vi "Fill Tree.vi"(8 "error in":errorcluster, 10 "Folder Path":path, 11 "TreeControl in":refnum<vi>) -> (0 "error out":errorcluster)   [LabVIEW 2019, in "SimpleDependencyInspector.lvlib" / "File Explorer.lvlib"]
uses:
  File Explorer.lvlib
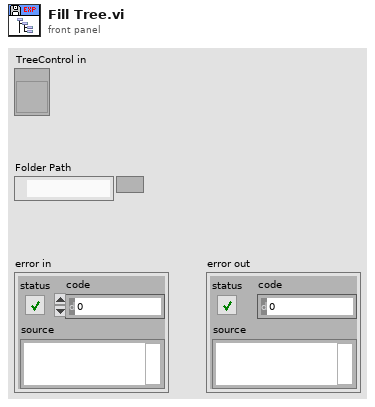
[diagram p1: front panel]
types:
  T1 = typedef "imagedata.ctl" = cluster{"image type":i32, "image depth":i32, "image":u8[], "mask":u8[], "colors":u32[], "Rectangle":cluster{"left":i16, "top":i16, "right":i16, "bottom":i16}}
  T2 = cluster{"Left Cell String":string, "Child Text":string[], "Child Tag":string, "Item Indent":i32, "Child Only?":bool, "Glyph Index":i32}[]
  T3 = cluster{"Left Cell String":string, "Child Text":string[], "Child Tag":string, "Item Indent":i32, "Child Only?":bool, "Glyph Index":i32}
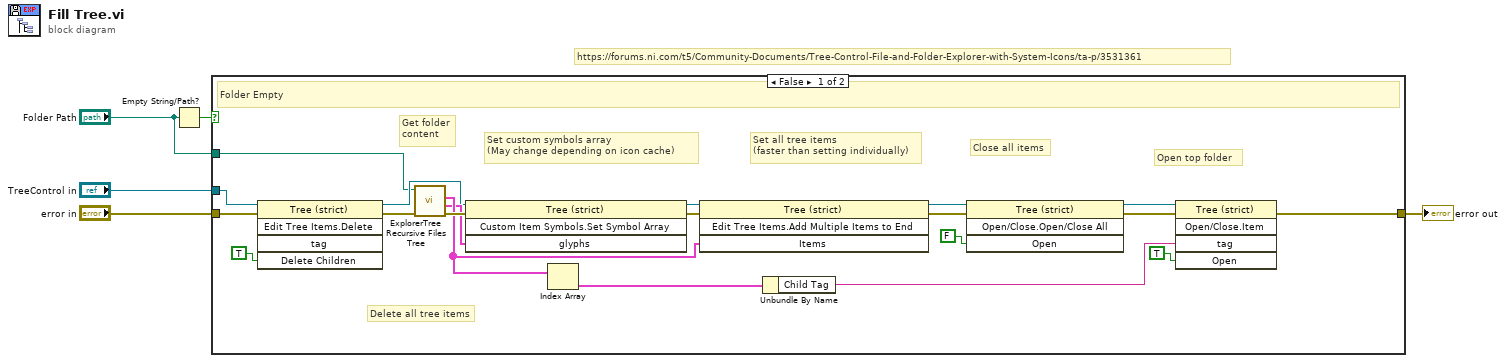
[diagram p0: block diagram]
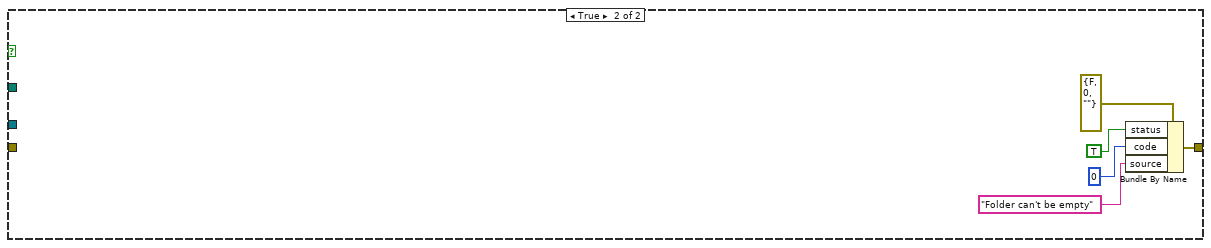
[diagram p2: hidden frame]
diagram:
  # "https://forums.ni.com/t5/Community-Documents/Tree-Control-File-and-Folder-Explorer-with-System-Icons/ta-p/3531361"
  n1 = Empty String/Path?(string/path="Folder Path") -> (empty?=w1:bool)
  n2 = case shown="False" w1 {
    tunnel: [w25 w29] -> w5
    tunnel: "error in" -> [w19 _]
    tunnel: "TreeControl in" -> [w7 _]
    tunnel: "Folder Path" -> [w6 _]
    frame False {
      # "Open top folder"
      # "Close all items"
      # "Set all tree items\n(faster than setting individually)"
      # "Set custom symbols array\n(May change depending on icon cache)"
      # "Get folder\ncontent"
      # "Delete all tree items"
      # "Folder Empty"
      n3 = invoke class="Tree (strict)" method="Edit Tree Items.Delete"(reference=w7, error in=w19, "Delete Children"=TRUE ("Delete Children?")) -> (reference out=w9:refnum<vi>, error out=w20:errorcluster)  [unwired: 2 in, 3 out]
      n4 = call "ExplorerTree Recursive Files Tree.vi"("error in (no error)"=w20, "Folder Path"=w6) -> ("error out"=w24:errorcluster, "Glyphs"=w10:T1[], "Items"=w15:T2)  [unwired: 6 in, 1 out]
      n5 = invoke class="Tree (strict)" method="Custom Item Symbols.Set Symbol Array"(reference=w9, error in=w24, "glyphs"=w10) -> (reference out=w11:refnum<vi>, error out=w21:errorcluster)  [unwired: 1 in, 2 out]
      n6 = Index Array(array=w15) -> (element=w16:T3)  [unwired: 1 in]
      n7 = invoke class="Tree (strict)" method="Edit Tree Items.Add Multiple Items to End"(reference=w11, error in=w21, "Items"=w15) -> (reference out=w12:refnum<vi>, error out=w22:errorcluster)  [unwired: 1 in, 2 out]
      n8 = Unbundle By Name(w16) -> ("Child Tag"=w17:string)
      n9 = invoke class="Tree (strict)" method="Open/Close.Open/Close All"(reference=w12, error in=w22, "Open"=FALSE ("Open?")) -> (reference out=w14:refnum<vi>, error out=w23:errorcluster)  [unwired: 1 in, 2 out]
      n10 = invoke class="Tree (strict)" method="Open/Close.Item"(reference=w14, error in=w23, "tag"=w17, "Open"=TRUE ("Open?")) -> (error out=w25:errorcluster)  [unwired: 1 in, 4 out]
    }
    frame True {
      n11 = Bundle By Name(cluster=errorcluster {"status"=FALSE, "code"=0, "source"=""} ("error constant"), "status"=TRUE, "code"=0, "source"="Folder can't be empty") -> (w29:errorcluster)
    }
  }
  "error out" <- w5
